vi "DimostratoreUpdateAutomation.vi"() -> ()   [LabVIEW 2019]
uses:
  ByteGSAPIBase.lvclass
  TypeDef/MachineStates.ctl
  TypeDef/Step.ctl
  TypeDef/Asset.ctl
panel:
  in  "Intruction Automation":string
  in  "Link Automation":string
  in  "Inizia Step":bool
  in  "Seleziona Step":i32(ring) items=["Plug and set the Power Supply"=36]
  out "Infos":string
  out "error out":errorcluster
  in  "error in (no error)":errorcluster
  in  "ByteGSAPIBase in":refnum<class "ByteGSAPIBase.lvclass">
  in  "Ottieni Passaggio Step":bool
  in  "Step Id":i32
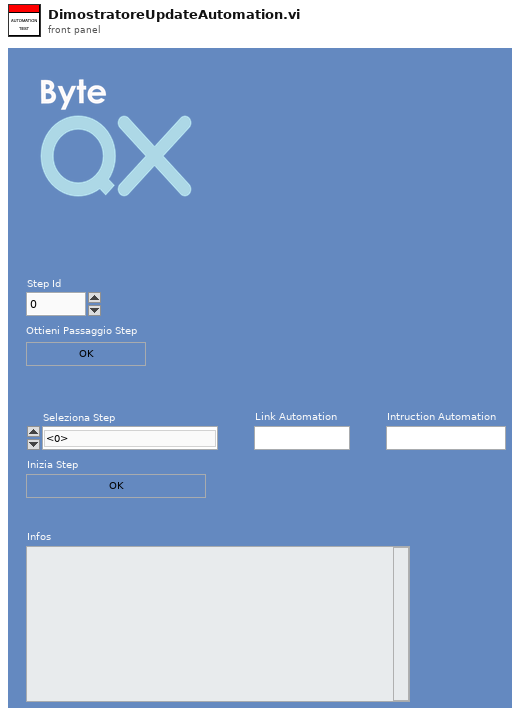
[diagram p1: front panel]
types:
  T1 = typedef "ByteGSWebAPI.lvlib/ByteGSAPIBase.lvclass/Step.ctl" = cluster{"id":i32, "descrizione":string, "prova":string, "assets":T2[], "criterio_accettazione":string, "valore_criterio_accettazione_max":dbl, "valore_criterio_accettazione_min":dbl, "udm_criterio_accettazione":string, "duration_prova":string, "udm_duration_prova":string, "valore_prova":dbl, "outcome":string, "ordine":i32, "user":i32, "link_automation":string, "instruction_automation":string, "data_completamento_checklist":timestamp}
  T2 = typedef "ByteGSWebAPI.lvlib/ByteGSAPIBase.lvclass/Asset.ctl" = cluster{"descrizione":string, "slug":string, "id":i32}
  T3 = typedef "MachineStates.ctl" = enum16{"Initialize", "Idle", "GetLimsTestsForBench", "AssetsCheck", "GetLimsTestSteps", "UpdateLimsTestStep", "GetLimsTestStep", "Indietro", "UpdateLimsTestStepAutomation"}
  T4 = cluster{"ByteGSAPIBase in":refnum<class "ByteGSAPIBase.lvclass">, "Steps Array":T1[]}
  T5 = cluster{"Step Id":i32, "Seleziona Step":i32, "Link Automation":string, "Intruction Automation":string}
  T6 = cluster{"duration_prova":string, "udm_duration_prova":string, "valore_prova":dbl, "outcome":string, "data_completamento_checklist":timestamp, "link_automation":string, "instruction_automation":string}
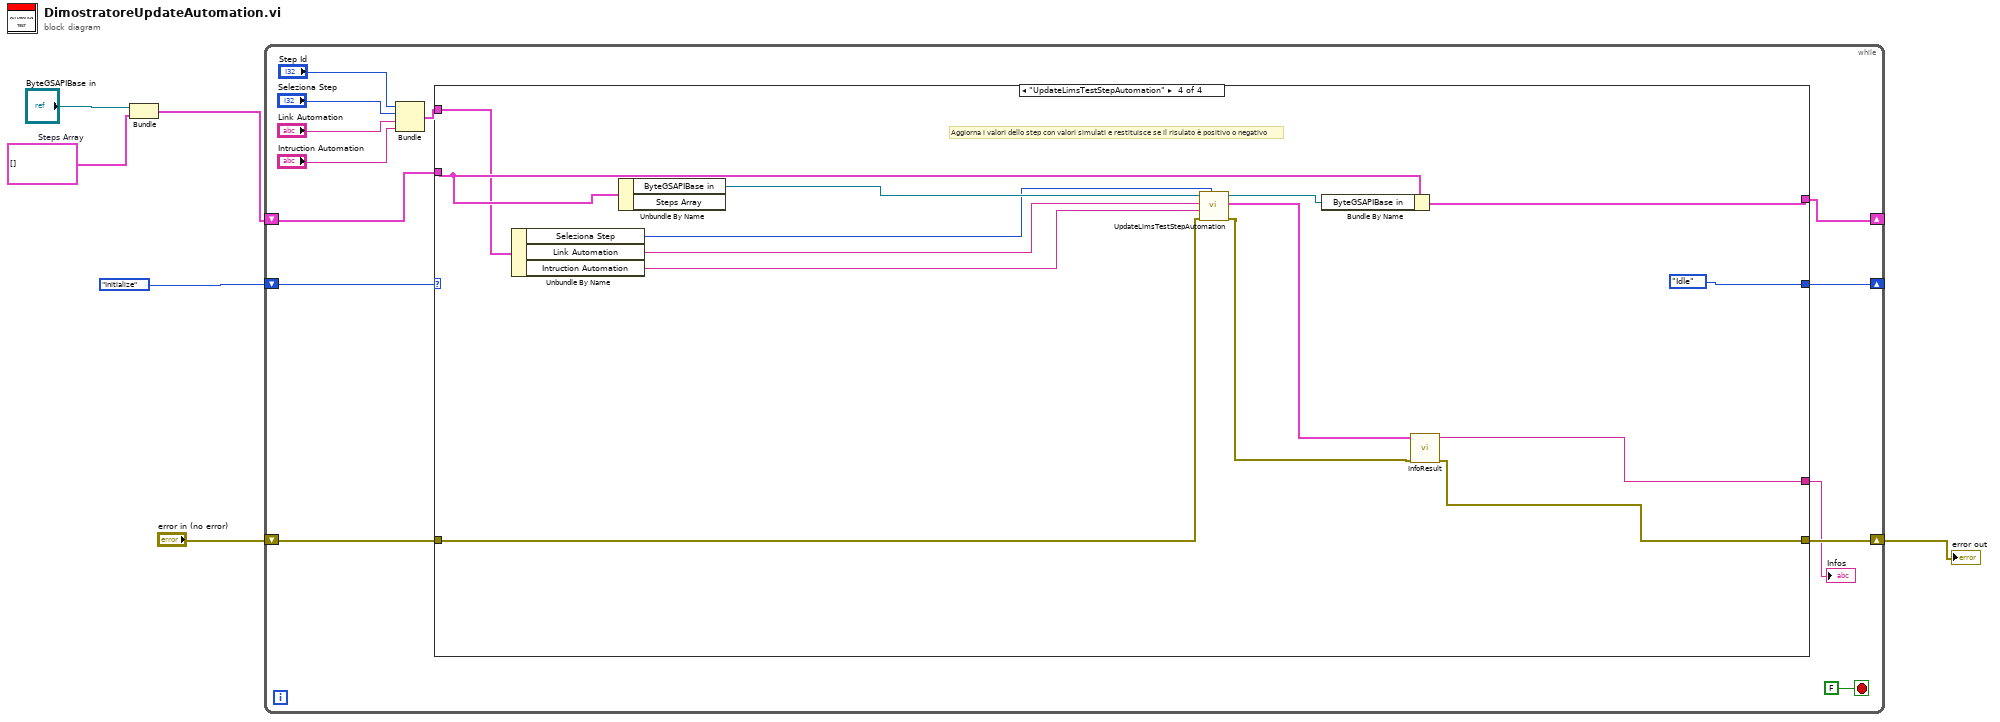
[diagram p0: block diagram]
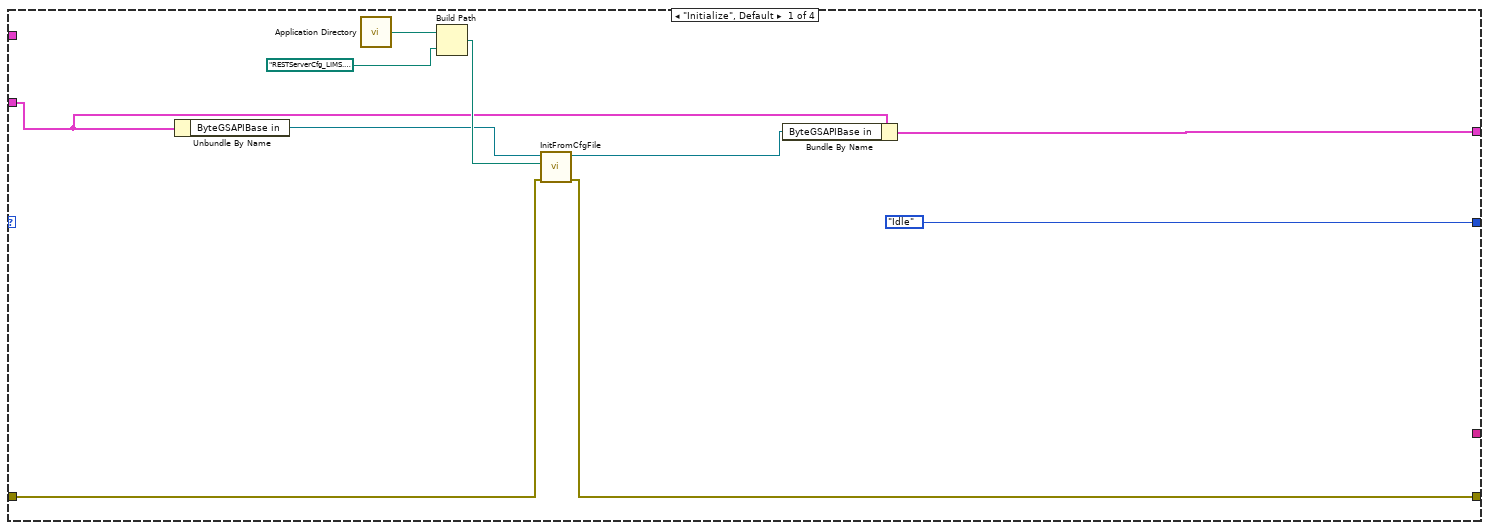
[diagram p2: hidden frame]
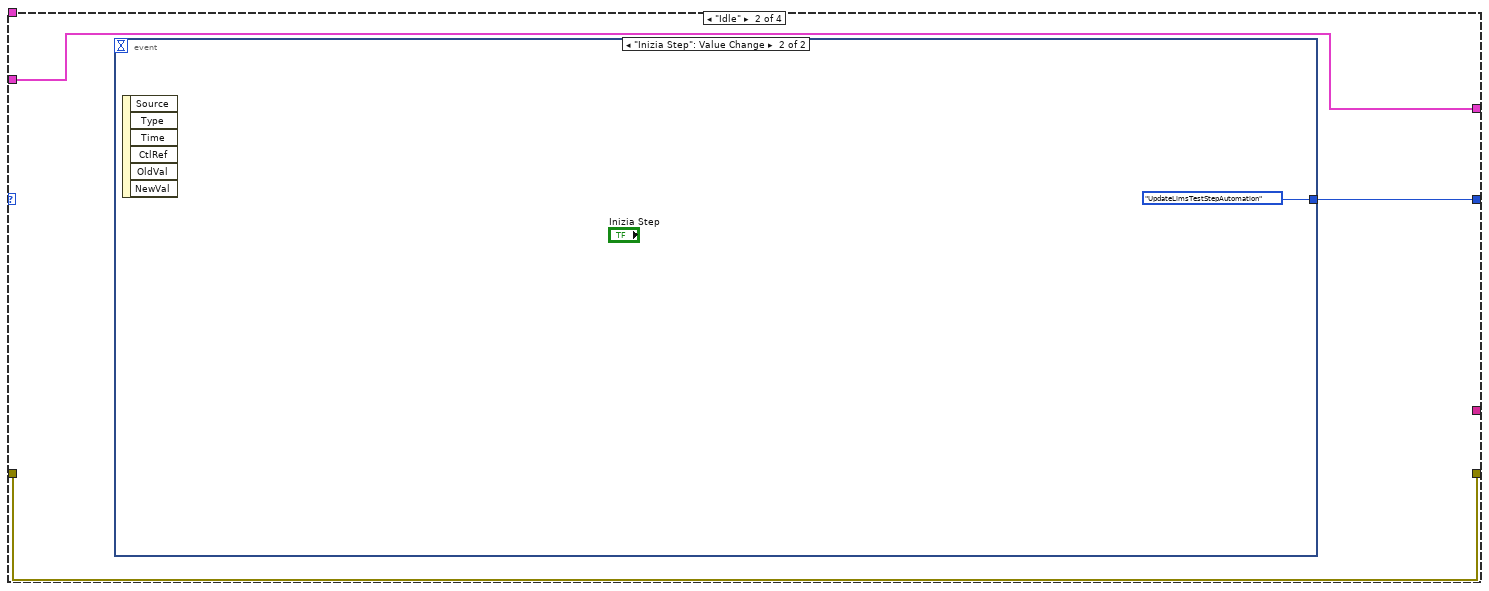
[diagram p3: hidden frame]
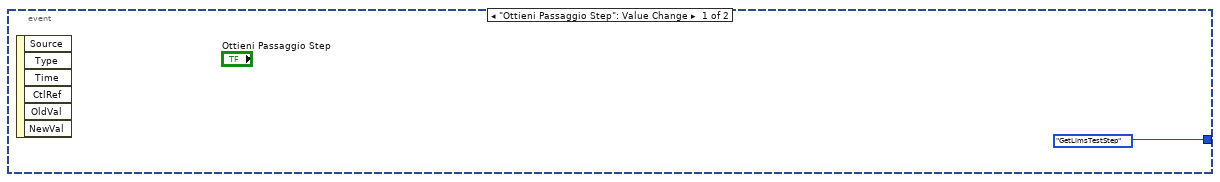
[diagram p4: hidden frame]
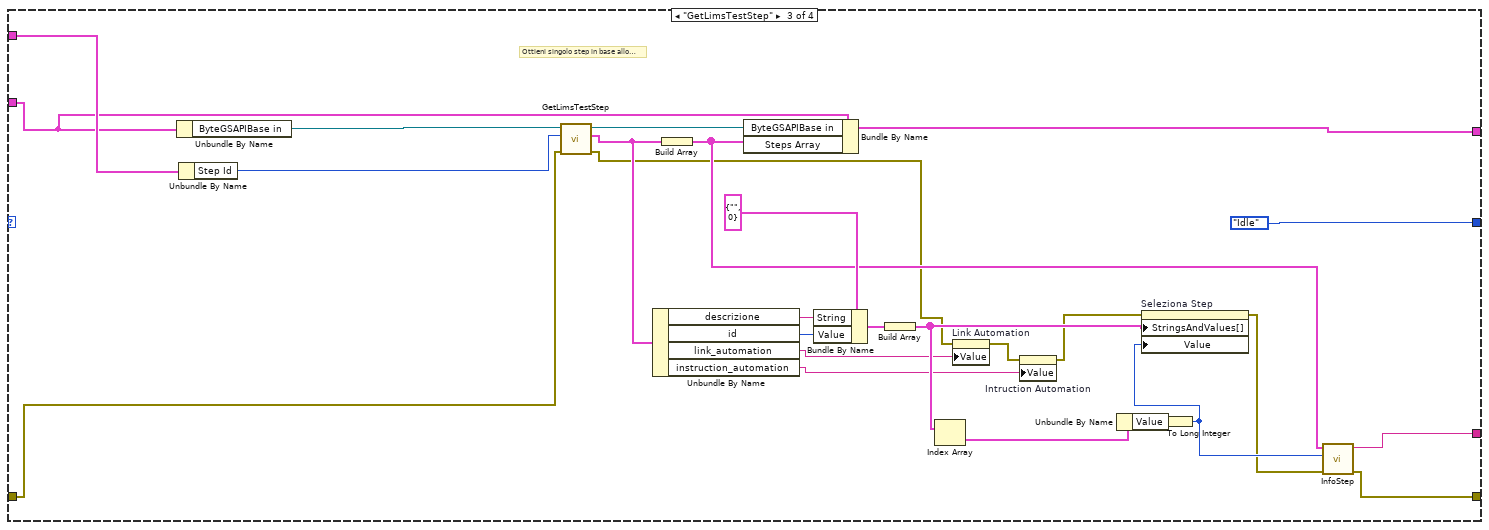
[diagram p5: hidden frame]
diagram:
  w4 = T1[] []  # Steps Array
  n1 = Bundle("ByteGSAPIBase in"="ByteGSAPIBase in", "Steps Array"=w4) -> (w3:T4)  [unwired: 1 in]
  n2 = while {
    shift-right: [w17] -> _
    shift-left: MachineStates."Initialize" ("Enum") -> [w19]
    shift-right: [w15] -> _
    shift-left: w3 -> [w16]
    shift-right: [w13] -> w1
    shift-left: "error in (no error)" -> [w14]
    stop <- FALSE stop-if-true
    n3 = Bundle("Step Id"="Step Id", "Seleziona Step"="Seleziona Step", "Link Automation"="Link Automation", "Intruction Automation"="Intruction Automation") -> (w11:T5)  [unwired: 1 in]
    n4 = case shown="\"UpdateLimsTestStepAutomation\"" w19 {
      tunnel: [MachineStates."Idle" ("Enum") w31 MachineStates."Idle" MachineStates."Idle"] -> w17
      tunnel: w16 -> [w23 w30 w47 w74]
      tunnel: [w22 w30 w46 w69] -> w15
      tunnel: w14 -> [w21 w32 w49 w66]
      tunnel: [w20 w32 w44 w71] -> w13
      tunnel: w11 -> [_ _ w48 w73]
      tunnel: [_ _ w45 w72] -> w10
      frame "Initialize", Default {
        n5 = Unbundle By Name(w23) -> ("ByteGSAPIBase in"=w26:refnum<class "ByteGSAPIBase.lvclass">)
        n6 = call <vilib>:"Application Directory.vi"() -> ("Application Directory"=w24:path)
        n7 = Build Path(base path=w24, name or relative path=path "RESTServerCfg_LIMS.ini") -> (appended path=w28:path)
        n8 = call-dynamic "InitFromCfgFile.vi"("error in (no error)"=w21, "configuration file path"=w28, "ByteGSAPIBase in"=w26) -> ("error out"=w20:errorcluster, "ByteGSAPIBase out"=w25:refnum<class "ByteGSAPIBase.lvclass">)  [unwired: 7 in]
        n9 = Bundle By Name(cluster=w23, "ByteGSAPIBase in"=w25) -> (w22:T4)
      }
      frame "Idle" {
        n10 = event shown="[1] \"Inizia Step\": Value Change" {
          selector: _ -> [_ _]
          dyn-events: _ -> [_ _]
          timeout: _ -> [_ _]
          tunnel: [MachineStates."GetLimsTestStep" ("Enum") MachineStates."UpdateLimsTestStepAutomation" ("Enum")] -> w31
          event "Ottieni Passaggio Step": Value Change {
            n11 = event-data() -> ()  [unwired: 1 in, 6 out]
          }
          event "Inizia Step": Value Change {
            n12 = event-data() -> ()  [unwired: 1 in, 6 out]
          }
        }
      }
      frame "GetLimsTestStep" {
        # "Ottieni singolo step in base allo step id"
        n13 = Unbundle By Name(w47) -> ("ByteGSAPIBase in"=w60:refnum<class "ByteGSAPIBase.lvclass">)
        n14 = Unbundle By Name(w48) -> ("Step Id"=w59:i32)
        n15 = call-dynamic "GetLimsTestStep.vi"("error in (no error)"=w49, "Step-id"=w59, "ByteGSAPIBase in"=w60) -> ("error out"=w37:errorcluster, "StepList"=w50:T1, "ByteGSAPIBase out"=w58:refnum<class "ByteGSAPIBase.lvclass">)  [unwired: 6 in]
        n16 = Unbundle By Name(w50) -> ("descrizione"=w55:string, "id"=w56:i32, "link_automation"=w39:string, "instruction_automation"=w38:string)
        n17 = Build Array(w50) -> (w51:T1[])
        n18 = Bundle By Name(cluster=w47, "ByteGSAPIBase in"=w58, "Steps Array"=w51) -> (w46:T4)
        n19 = Bundle By Name(cluster=cluster{"String":string, "Value":u16} {"String"="", "Value"=0} ("Cluster"), "String"=w55, "Value"=w56) -> (w53:cluster{"String":string, "Value":u16})
        n20 = Build Array(w53) -> (w43:cluster{"String":string, "Value":u16}[])
        n21 = Index Array(array=w43) -> (element=w57:cluster{"String":string, "Value":u16})  [unwired: 1 in]
        n22 = property on="Link Automation" class="Str"(error in=w37, "Value"=w39) -> (error out=w36:errorcluster)  [unwired: 1 in, 1 out]
        n23 = property on="Intruction Automation" class="Str"(error in=w36, "Value"=w38) -> (error out=w35:errorcluster)  [unwired: 1 in, 1 out]
        n24 = Unbundle By Name(w57) -> ("Value"=w52:u16)
        n25 = To Long Integer(number=w52) -> (32bit integer=w42:i32)
        n26 = property on="Seleziona Step" class="Ring (strict)"(error in=w35, "StringsAndValues[]"=w43, "Value"=w42) -> (error out=w41:errorcluster)  [unwired: 1 in, 1 out]
        n27 = call "InfoStep.vi"("error in"=w41, "Seleziona Step"=w42, "Test Steps List"=w51) -> ("error out"=w44:errorcluster, "Info Test"=w45:string)  [unwired: 7 in]
      }
      frame "UpdateLimsTestStepAutomation" {
        # "Aggiorna i valori dello step con valori simulati e restituisce se il risulato è positivo o negativo"
        n28 = Unbundle By Name(w73) -> ("Seleziona Step"=w63:i32, "Link Automation"=w62:string, "Intruction Automation"=w61:string)
        n29 = Unbundle By Name(w74) -> ("ByteGSAPIBase in"=w68:refnum<class "ByteGSAPIBase.lvclass">)  [unwired: 1 out]
        n30 = call "UpdateLimsTestStepAutomation.vi"("step_id"=w63, "error in (no error)"=w66, "instruction_automation"=w61, "link_automation"=w62, "ByteGSAPIBase in"=w68) -> ("error out"=w67:errorcluster, "Result Step"=w65:T6, "ByteGSAPIBase out"=w64:refnum<class "ByteGSAPIBase.lvclass">)  [unwired: 4 in]
        n31 = Bundle By Name(cluster=w74, "ByteGSAPIBase in"=w64) -> (w69:T4)
        n32 = call "InfoResult.vi"("error in"=w67, "Result Step"=w65) -> ("error out"=w71:errorcluster, "Info Test"=w72:string)  [unwired: 8 in]
      }
    }
    "Infos" <- w10
  }
  "error out" <- w1
